vi "Alazar_SetRecord -ATS-SDK.vi"(8 "error in (no error)":errorcluster, 9 "Pts to Acquire":u32, 10 "Records":u32=1, 11 "Handle":u32) -> (0 "error out":errorcluster, 1 "Return Code":u32, 2 "RecordOut":T1={"Count"=1, "Presize"=1, "Length"=0}, 3 "Handle Out":u32)   [LabVIEW 2022 SP3]
doc: "_____AlazarTech, Scope_____\n\nConfigure the number of records for the device to capture."
uses:
  Record.ctl
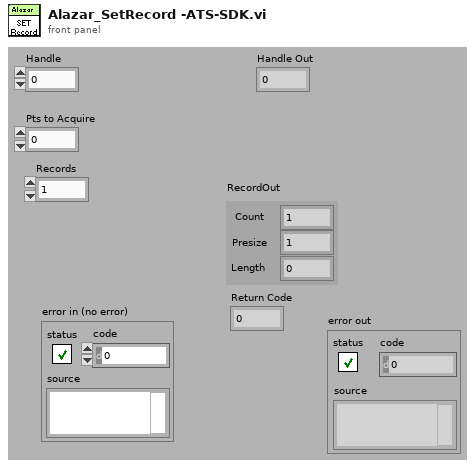
[diagram p1: front panel]
types:
  T1 = typedef "Record.ctl" = cluster{"Count":u32, "Presize":u32, "Length":u32}
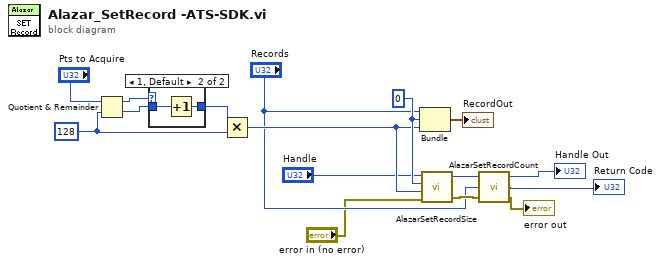
[diagram p0: block diagram]
diagram:
  w16 = u32 128 ("y")
  w13 = u32 0 ("Count")
  n1 = Quotient & Remainder(x="Pts to Acquire", y=w16) -> (x-y*floor(x/y)=w3:u32, floor(x/y)=w2:u32)
  n2 = case shown="1, Default" w3 {
    tunnel: [w17 w19] -> w1
    tunnel: w2 -> [w17 w18]
    frame 0 {
    }
    frame 1, Default {
      n3 = Increment(x=w18) -> (x+1=w19:u32)
    }
  }
  n4 = Multiply(x=w1, y=w16) -> (x*y=w12:u32)
  n5 = Bundle("Records"="Records", "Count"=w13, w12) -> (→"RecordOut":cluster{"Records":u32, "Count":u32, u32})  [unwired: 1 in]
  n6 = call "AlazarSetRecordSize.vi"("error in (no error)"="error in (no error)", "Post-trigger Samples"=w12, "Pre-trigger Samples"=w13, "Handle"="Handle") -> ("error out"=w10:errorcluster, "Handle"=w11:u64)  [unwired: 1 out]
  n7 = call "AlazarSetRecordCount.vi"("error in (no error)"=w10, "Count"="Records", "Handle"=w11) -> ("error out"=→"error out":errorcluster, "Return Code"=→"Return Code":u32, "Handle"=→"Handle Out":u64)
